vi "Demo1-Basic_Queries.vi"() -> ()   [LabVIEW 2020]
panel:
  out "(For your Reference:)\nKeyword Description":string
  in  "IP Address of Remote Device":string="196.254.31.200"
  in  "Disconnect":bool
  out "(For your Reference: )\n Query Sent to Device":string
  out "Device Response to Query":string
  in  "SCPI-Style Keyword":u16(ring) items=["*IDN", "TRIGger:COUNt", "TRIGger:DECimation", "SYSTem:TIME", "SYSTem:TIME:UNIX", "MCU:TEMPerature", "DIODe:TRACe:DT", "DIODe:TRACe:NT", "DIODe:TRACe:YMIN", "DIODe:TRACe:YMAX", "DIODe:METRics:SIZE", "DIODe:DT", "DIODe:T1:VALue", "DIODe:T2:VALue", "DIODe:T2:NT", "DIODe:T3:VALue", "DIODe:T3:NT", "DIODe:T4:VALue", "DIODe:T4:NT"]
  # "Diode Demo - Basic Queries"
  # "Demonstrates simple queries to the STM32 Diode Device."
  # "VI Instructions\n\n1. Make sure you know the Device IP Address.\n2. From Windows command prompt, confirm ping to IP address.\n3. Type the correct device IP address into this VI.\n3. Run this VI.\n4. While running, select various SCPI-Style Keywords from the dropdown menu and observe device responses.\n5. When finished exploring queries, disconnect safely from the device via the \"Disconnect\" toggle button. (Not the Abort button).\n\nCreated by Scott Feister on July 13, 2022."
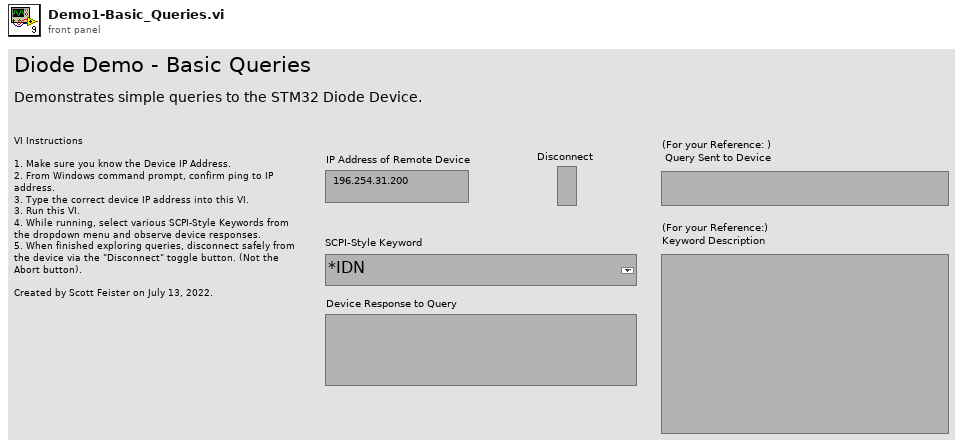
[diagram p1: front panel]
types:
  T1 = typedef "DDAQ-Keyword.ctl" = cluster{"Keyword":string, "Gettable":bool, "Settable":bool, "Is Array":bool, "Data Type":string, "Description":string}
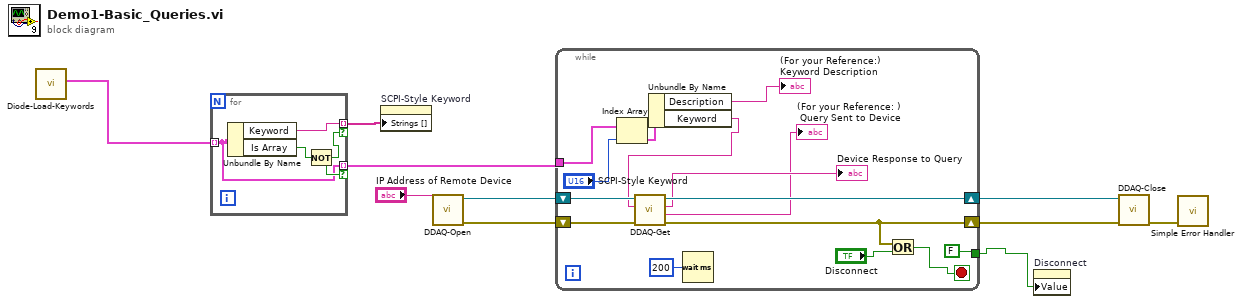
[diagram p0: block diagram]
diagram:
  n1 = call "Diode-Load-Keywords.vi"() -> ("Diodes Keywords Array"=w2:T1[])  [unwired: 11 in]
  n2 = for {
    tunnel: w2 -> [w11] mode=indexing
    tunnel: [w14] -> w5 mode=indexing if=w12
    tunnel: [w11] -> w1 mode=indexing if=w12
    n3 = Unbundle By Name(w11) -> ("Keyword"=w14:string, "Is Array"=w13:bool)
    n4 = Not(x=w13) -> (.not. x?=w12:bool)
  }
  n5 = property on="SCPI-Style Keyword" class="Ring (strict)"("Strings []"=w5) -> ()  [unwired: 2 in, 2 out]
  n6 = call "DDAQ-Open.vi"("IP Address of Nucleo Device"="IP Address of Remote Device") -> ("error out"=w9:errorcluster, "connection ID"=w10:refnum<k5>)  [unwired: 8 in, 1 out]
  n7 = while {
    shift-right: [w27] -> w8
    shift-left: w10 -> [w29]
    shift-right: [w20] -> w7
    shift-left: w9 -> [w28]
    tunnel: w1 -> [w24]
    tunnel: [FALSE] -> w4
    stop <- w19 stop-if-true
    n8 = Index Array(array=w24, index="SCPI-Style Keyword") -> (element=w18:T1)
    n9 = Unbundle By Name(w18) -> ("Description"=→"(For your Reference:)\nKeyword Description":string, "Keyword"=w15:string)
    n10 = call "DDAQ-Get.vi"("error in (no error)"=w28, "SCPI-like Keyword (leave off question mark)"=w15, "connection ID"=w29) -> ("error out"=w20:errorcluster, "Query"=→"(For your Reference: )\n Query Sent to Device":string, "Response"=→"Device Response to Query":string, "connection ID out"=w27:refnum<k5>)  [unwired: 4 in, 1 out]
    n11 = Wait (ms)(milliseconds to wait=u32 200) -> ()  [unwired: 1 out]
    n12 = Or(x=w20, y="Disconnect") -> (x .or. y?=w19:bool)
  }
  n13 = property on="Disconnect" class="Bool (strict)"("Value"=w4) -> ()  [unwired: 2 in, 2 out]
  n14 = call "DDAQ-Close.vi"("error in (no error)"=w7, "connection ID"=w8) -> ("error out"=w6:errorcluster)  [unwired: 8 in, 1 out]
  n15 = call <vilib>:"Simple Error Handler.vi"("error in (no error)"=w6) -> ()  [unwired: 4 in, 5 out]
